vi "Delay Integer.vi"(2 "Enum":T1(ring), 5 "input":i32, 9 "Delay":i32) -> (6 "Output":i32, 8 "Debounced":dbl, 10 "History":i32[](array[numeric]))   [LabVIEW 2016]
doc: "Every milisecond this VI inserts the value of the input terminal into an array at an index equal to delay pushing every other value in the array one index toward zero. The output terminal is equal to the zero index of the array. The array can be retrived from the history terminal and the average of the array can be retrived from the debounced terminal.\n\nThe mode terminal sets the mode of the delay. when the mode is set to falling the VI reinitializes the entire array as true when the button is pressed. In falling mode it reintitializes it as false when the button is released. Neither mode will not reinitalize when the input changes. Instant mode will remove the milisecond wait and complete all of the tasks once per cycle.\n\nWhen the Value of the delay terminal is changed the array is reinitialized as false.\n\nWhen the boolean polymorphic subVI recives true on the invert terminal it inverts it's input and all array initializations/reinitializations.\n\nWhen the doubble or integer polymorphic subVI is set to falling mode it sends the input directly to the output until it is set to zero. when set to zero it will send the last non zero value for delay ms. Rising mode does the opposite. \n\nCreated by Team 4130 for use in the 2016-2017 FRC season"
uses:
  <vilib>/Analysis/baseanly.llb/Mean (DBL).vi
  <vilib>/Analysis/NI_AALBase.lvlib
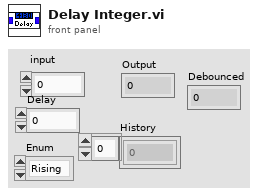
[diagram p1: front panel]
types:
  T1 = enum16{"Rising", "Falling", "Neither", "Instant"}
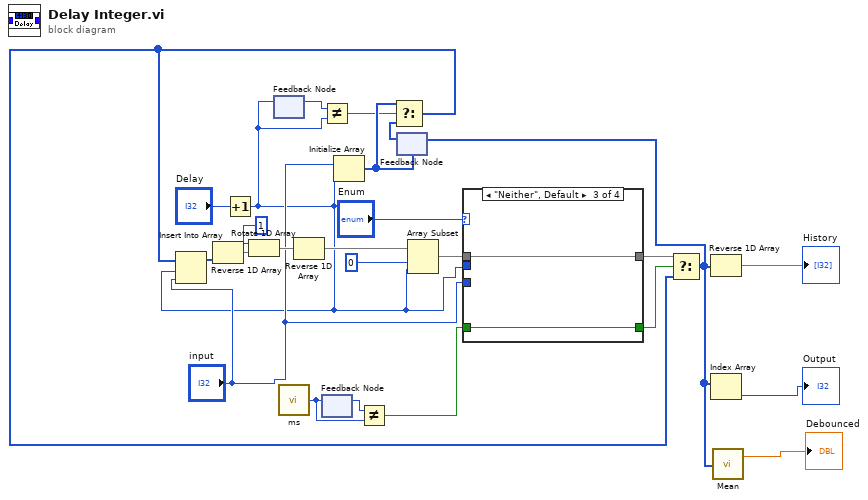
[diagram p0: block diagram]
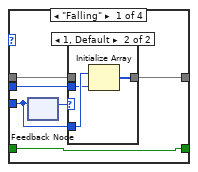
[diagram p2: hidden frame]
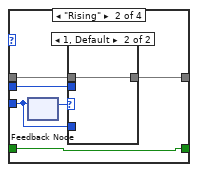
[diagram p4: hidden frame]
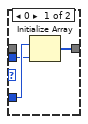
[diagram p5: hidden frame]
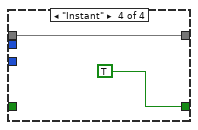
[diagram p6: hidden frame]
diagram:
  n1 = Increment(x="Delay") -> (x+1=w2:i32)
  n2 = feedback #1() -> (w12:i32)  [unwired: 1 in]
  n3 = feedback-in #1(w2) -> ()
  n4 = call "ms.vi"() -> ("millisecond"=w24:u32)  [unwired: 1 in]
  n5 = Not Equal?(x=w12, y=w2) -> (x != y?=w11:bool)
  n6 = feedback #2() -> (w25:u32)  [unwired: 1 in]
  n7 = feedback-in #2(w24) -> ()
  n8 = Initialize Array("input", w2) -> (w14:i32[])
  n9 = Not Equal?(x=w25, y=w24) -> (x != y?=w1:bool)
  n10 = feedback #3(w14) -> (w13:i32[])
  n11 = Select(t=w14, s=w11, f=w13) -> (s? t:f=w8:i32[])
  n12 = Insert Into Array(array=w8, index=w2, new element="input") -> (w9:i32[])
  n13 = Reverse 1D Array(array=w9) -> (reversed array=w21:i32[])
  n14 = Rotate 1D Array(1:w21, 2:1 ("n")) -> (0:w23:i32[])
  n15 = Reverse 1D Array(array=w23) -> (reversed array=w10:i32[])
  n16 = Array Subset(array=w10, index=0, length=w2) -> (w17:i32[])
  n17 = case shown="\"Neither\", Default" "Enum" {
    tunnel: w17 -> [w29 w39 w47 w49]
    tunnel: [w31 w41 w47 w49] -> w20
    tunnel: "input" -> [w28 w38 _ _]
    tunnel: w2 -> [w30 w40 _ _]
    tunnel: [w26 w36 w46 TRUE] -> w18
    tunnel: w1 -> [w26 w36 w46 _]
    frame "Falling" {
      n18 = feedback-in #4(w28) -> ()
      n19 = feedback #4() -> (w27:i32)  [unwired: 1 in]
      n20 = case shown="1, Default" w27 {
        tunnel: [w32 w35] -> w31
        tunnel: w28 -> [_ w34]
        tunnel: w30 -> [_ w33]
        tunnel: w29 -> [w32 _]
        frame 0 {
        }
        frame 1, Default {
          n21 = Initialize Array(w34, w33) -> (w35:i32[])
        }
      }
    }
    frame "Rising" {
      n22 = feedback-in #5(w38) -> ()
      n23 = feedback #5() -> (w37:i32)  [unwired: 1 in]
      n24 = case shown="1, Default" w37 {
        tunnel: [w44 w45] -> w41
        tunnel: w38 -> [w43 _]
        tunnel: w40 -> [w42 _]
        tunnel: w39 -> [_ w45]
        frame 0 {
          n25 = Initialize Array(w43, w42) -> (w44:i32[])
        }
        frame 1, Default {
        }
      }
    }
    frame "Neither", Default {
    }
    frame "Instant" {
    }
  }
  n26 = Select(t=w20, s=w18, f=w8) -> (s? t:f=w15:i32[])
  n27 = feedback-in #3(w15) -> ()
  n28 = Reverse 1D Array(array=w15) -> (reversed array=→"History":i32[])
  n29 = Index Array(array=w15) -> (element=→"Output":i32)  [unwired: 1 in]
  n30 = call-poly <vilib>:"Mean.vi"("X"=w15) -> ("mean"=→"Debounced":dbl)  [unwired: 1 out]
